vi "Webview_Init.vi"(4 "Environment Options":T1, 6 "Path Overrides":T2, 8 "Error In":errorcluster, 10 "WebView2 Control in":refnum<k24>(container), 11 "object in":refnum<class "WebView.lvclass">) -> (0 "Error Out":errorcluster, 3 "object out":refnum<class "WebView.lvclass">)   [LabVIEW 2024, in "WebView.lvclass"]
uses:
  WebView.lvclass
  Paths-cluster.ctl
  Core Envrionment Options--cluster.ctl
  <vilib>/sklein/WebView2/Libs/Microsoft.Web.WebView2.WinForms.dll
  WebView.lvclass/WebView.ctl
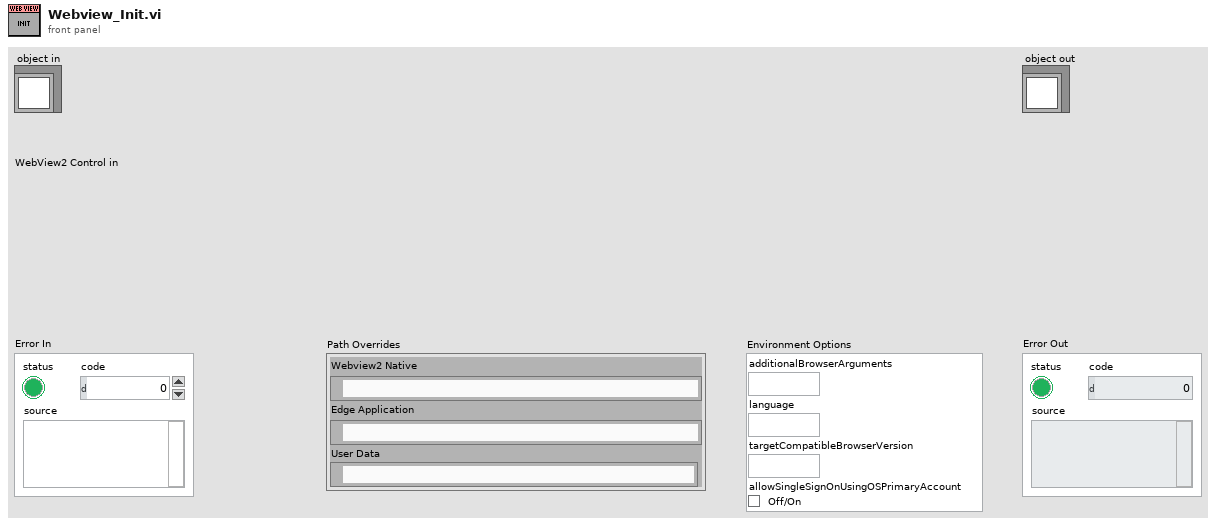
[diagram p1: front panel]
types:
  T1 = typedef "WebView.lvclass/Core Envrionment Options--cluster.ctl" = cluster{"additionalBrowserArguments":string, "language":string, "targetCompatibleBrowserVersion":string, "allowSingleSignOnUsingOSPrimaryAccount":bool}
  T2 = typedef "WebView.lvclass/Paths-cluster.ctl" = cluster{"Webview2 Native":path, "Edge Application":path, "User Data":path}
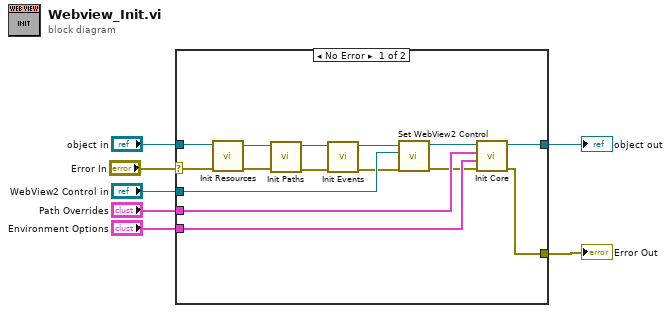
[diagram p0: block diagram]
diagram:
  n1 = case shown="No Error" "Error In" {
    selector: "Error In" -> [w15 w23]
    tunnel: "object in" -> [w22 w24]
    tunnel: [w21 w24] -> w6
    tunnel: [w20 w23] -> w4
    tunnel: "Path Overrides" -> [w18 _]
    tunnel: "Environment Options" -> [w19 _]
    tunnel: "WebView2 Control in" -> [w14 _]
    frame No Error {
      n2 = call "Init Resources.vi"("Error In"=w15, "WebView in"=w22) -> ("Error Out"=w12:errorcluster, "WebView out"=w13:refnum<class "WebView.lvclass">)  [unwired: 8 in]
      n3 = call "Init Paths.vi"("Error In"=w12, "WebView in"=w13) -> ("Error Out"=w10:errorcluster, "WebView out"=w11:refnum<class "WebView.lvclass">)  [unwired: 8 in]
      n4 = call "Init Events.vi"("Error In"=w10, "WebView in"=w11) -> ("Error Out"=w8:errorcluster, "WebView out"=w9:refnum<class "WebView.lvclass">)  [unwired: 8 in]
      n5 = call "Set WebView2 Control.vi"("Error In"=w8, "WebView2 Control"=w14, "object in"=w9) -> ("Error Out"=w16:errorcluster, "object out"=w17:refnum<class "WebView.lvclass">)  [unwired: 7 in]
      n6 = call "Init Core.vi"("Error In"=w16, "Environment Options"=w19, "Path Overrides"=w18, "object in"=w17) -> ("Error Out"=w20:errorcluster, "object out"=w21:refnum<class "WebView.lvclass">)  [unwired: 6 in]
    }
    frame Error {
    }
  }
  "object out" <- w6
  "Error Out" <- w4
